vi "BMark_Create Tree.vi"(7 "Bookmarks":T2[](array[typedef]), 8 "Error In":errorcluster, 10 "Bookmarks Grouping":T1, 11 "Bookmarks View In":refnum<vi>) -> (0 "Error Out":errorcluster, 3 "Bookmarks View Out":refnum<vi>)   [LabVIEW 2018, in "Bookmark Manager.lvlib"]
uses:
  Bookmark Manager.lvlib
  Controls/BMark_Bookmark Data.ctl
  Controls/BMark_VI_Identifier.ctl
  <vilib>/addons/analyzer/_analyzerctrls.llb/VIAnCtl Analysis App Info.ctl
  Controls/Bookmarks Groups.ctl
  Toolkit/Typedefs/Bookmark Tags.ctl
  Toolkit/Toolkit.lvlib
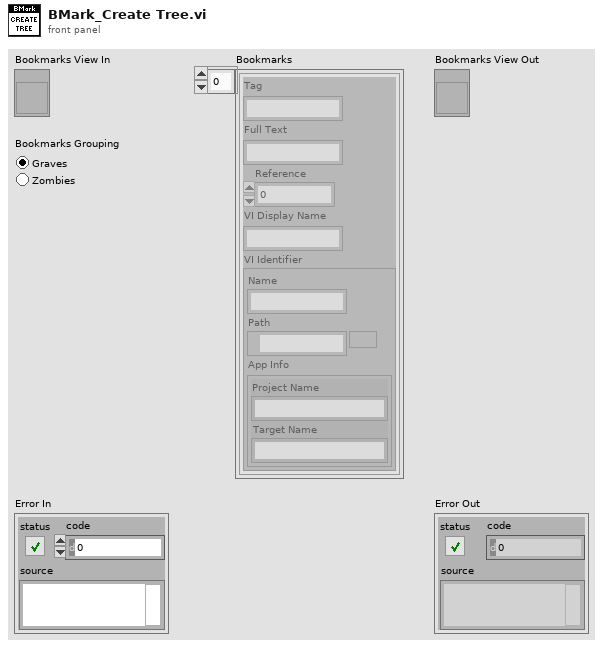
[diagram p1: front panel]
types:
  T1 = typedef "Bookmark Manager.lvlib/Bookmarks Groups.ctl" = enum32{"Graves", "Zombies"}
  T2 = typedef "Bookmark Manager.lvlib/BMark_Bookmark Data.ctl" = cluster{"Tag":string, "Full Text":string, "Reference":i32, "VI Display Name":string, "VI Identifier":T3}
  T3 = typedef "Bookmark Manager.lvlib/BMark_VI_Identifier.ctl" = cluster{"Name":string, "Path":path, "App Info":T4}
  T4 = typedef "VIAnCtl Analysis App Info.ctl" = cluster{"Project Name":string, "Target Name":string}
  T5 = enum8{"Enabled", "Disabled", "Disabled and Grayed Out"}
  T6 = typedef "Toolkit.lvlib/Bookmark Tags.ctl" = enum16{"RIP", "Zombie"}
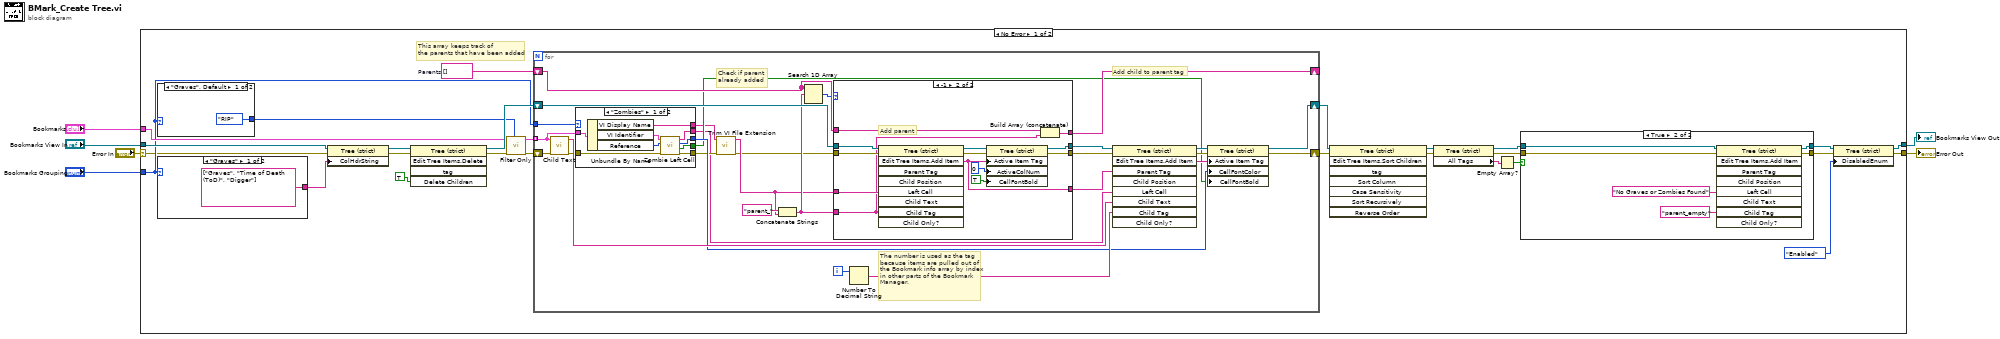
[diagram p0: block diagram]
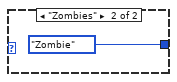
[diagram p2: hidden frame]
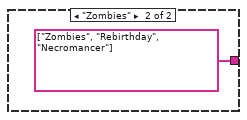
[diagram p3: hidden frame]
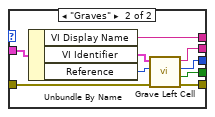
[diagram p4: hidden frame]
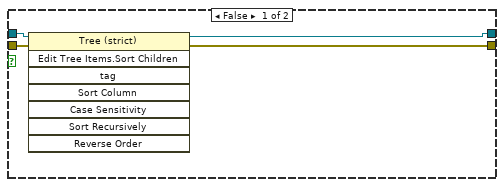
[diagram p6: hidden frame]
diagram:
  n1 = case shown="No Error" "Error In" {
    selector: "Error In" -> [w7 w112]
    tunnel: "Bookmarks View In" -> [w27 w111]
    tunnel: [w17 w112] -> w5
    tunnel: [w15 w111] -> w4
    tunnel: "Bookmarks" -> [w13 _]
    tunnel: "Bookmarks Grouping" -> [w8 _]
    frame No Error {
      w31 = string[] []  # Parents
      # "This array keeps track of \nthe parents that have been added"
      n2 = case shown="\"Graves\", Default" w8 {
        tunnel: [Bookmark_Tags."RIP" ("Bookmark") Bookmark_Tags."Zombie" ("Bookmark")] -> w12
        frame "Graves", Default {
        }
        frame "Zombies" {
        }
      }
      n3 = case shown="\"Graves\"" w8 {
        tunnel: [string[] ["Graves", "Time of Death (ToD)", "Digger"] string[] ["Zombies", "Rebirthday", "Necromancer"]] -> w14
        frame "Graves" {
        }
        frame "Zombies" {
        }
      }
      n4 = property class="Tree (strict)"(reference=w27, error in=w7, "ColHdrString"=w14) -> (reference out=w25:refnum<vi>, error out=w26:errorcluster)
      n5 = invoke class="Tree (strict)" method="Edit Tree Items.Delete"(reference=w25, error in=w26, "Delete Children"=TRUE ("Delete Children?")) -> (reference out=w32:refnum<vi>, error out=w11:errorcluster)  [unwired: 2 in, 3 out]
      n6 = call "Filter Only.vi"("Bookmark"=w12, "Error In"=w11, "All Bookmarks"=w13) -> ("Error Out"=w10:errorcluster, "Filtered Bookmarks"=w9:T2[])  [unwired: 7 in]
      n7 = for {
        tunnel: w9 -> [w52] mode=indexing
        shift-right: [w64] -> _
        shift-left: w31 -> [w65]
        shift-right: [w48] -> w30
        shift-left: w32 -> [w63]
        tunnel: w8 -> [w56]
        shift-right: [w46] -> w16
        shift-left: w10 -> [w51]
        i -> [w54]
        # "The number is used as the tag because items are pulled out of the Bookmark info array by index in other parts of the Bookmark Manager."
        # "Check if parent\nalready added"
        # "Add child to parent tag"
        n8 = call "Child Text.vi"("Error In"=w51, "Bookmark"=w52) -> ("Error Out"=w49:errorcluster, "Child Text"=w50:string[])  [unwired: 8 in]
        n9 = case shown="\"Zombies\"" w56 {
          tunnel: w52 -> [w74 w81]
          tunnel: [w73 w83] -> w39
          tunnel: [w68 w75] -> w38
          tunnel: w49 -> [w72 w82]
          tunnel: [w69 w78] -> w41
          tunnel: [w67 w76] -> w44
          tunnel: [w66 w77] -> w43
          frame "Zombies" {
            n10 = Unbundle By Name(w74) -> ("VI Display Name"=w73:string, "VI Identifier"=w71:T3, "Reference"=w70:i32)
            n11 = call "Zombie Left Cell.vi"("Error In"=w72, "Bookmark ID"=w70, "VI Identifier"=w71) -> ("Error Out"=w69:errorcluster, "Bold?"=w66:bool, "Color"=w67:u32, "Text"=w68:string)  [unwired: 5 in]
          }
          frame "Graves" {
            n12 = Unbundle By Name(w81) -> ("VI Display Name"=w83:string, "VI Identifier"=w80:T3, "Reference"=w79:i32)
            n13 = call "Grave Left Cell.vi"("Error In"=w82, "Bookmark ID"=w79, "VI Identifier"=w80) -> ("Error Out"=w78:errorcluster, "Bold?"=w77:bool, "Color"=w76:u32, "Text"=w75:string)  [unwired: 5 in]
          }
        }
        n14 = call "Trim VI File Extension.vi"("Error In"=w41, "VI File Name"=w39) -> ("Error Out"=w40:errorcluster, "VI Name"=w42:string)  [unwired: 8 in]
        n15 = Concatenate Strings("parent_", w42) -> (w58:string)
        n16 = Search 1D Array(1D array=w65, element=w58) -> (index of element=w55:i32)  [unwired: 1 in]
        n17 = case shown="-1" w55 {
          tunnel: w65 -> [w87 w100]
          tunnel: w58 -> [w84 w93]
          tunnel: [w87 w99] -> w64
          tunnel: w40 -> [w85 w97]
          tunnel: [w85 w90] -> w57
          tunnel: w63 -> [w86 w98]
          tunnel: [w86 w89] -> w62
          tunnel: [w84 w88] -> w61
          tunnel: w42 -> [_ w96]
          frame Default {
            # "Tag previously added"
          }
          frame -1 {
            # "Add parent"
            n18 = invoke class="Tree (strict)" method="Edit Tree Items.Add Item"(reference=w98, error in=w97, "Left Cell"=w96, "Child Tag"=w93) -> (reference out=w95:refnum<vi>, error out=w94:errorcluster, "Edit Tree Items:Add Item"=w88:string)  [unwired: 5 in, 6 out]
            n19 = property class="Tree (strict)"(reference=w95, error in=w94, "Active Item Tag"=w88, "ActiveColNum"=0 ("Active Cell:Active Column Number"), "CellFontBold"=TRUE ("Active Cell:Cell Font:Bold")) -> (reference out=w89:refnum<vi>, error out=w90:errorcluster)
            n20 = Build Array (concatenate)(w100, w93) -> (w99:string[])
          }
        }
        n21 = Number To Decimal String(number=w54) -> (decimal integer string=w53:string)  [unwired: 1 in]
        n22 = invoke class="Tree (strict)" method="Edit Tree Items.Add Item"(reference=w62, error in=w57, "Parent Tag"=w61, "Left Cell"=w38, "Child Text"=w50, "Child Tag"=w53) -> (reference out=w59:refnum<vi>, error out=w47:errorcluster, "Edit Tree Items:Add Item"=w45:string)  [unwired: 3 in, 6 out]
        n23 = property class="Tree (strict)"(reference=w59, error in=w47, "Active Item Tag"=w45, "CellFontColor"=w44, "CellFontBold"=w43) -> (reference out=w48:refnum<vi>, error out=w46:errorcluster)
      }
      n24 = invoke class="Tree (strict)" method="Edit Tree Items.Sort Children"(reference=w30, error in=w16) -> (reference out=w24:refnum<vi>, error out=w23:errorcluster)  [unwired: 6 in, 6 out]
      n25 = property class="Tree (strict)"(reference=w24, error in=w23) -> (reference out=w29:refnum<vi>, error out=w28:errorcluster, "All Tags"=w22:string[])
      n26 = Empty Array?(array=w22) -> (empty?=w21:bool)
      n27 = case shown="True" w21 {
        tunnel: w29 -> [w104 w110]
        tunnel: w28 -> [w103 w109]
        tunnel: [w102 w108] -> w19
        tunnel: [w101 w106] -> w20
        frame False {
          n28 = invoke class="Tree (strict)" method="Edit Tree Items.Sort Children"(reference=w104, error in=w103) -> (reference out=w101:refnum<vi>, error out=w102:errorcluster)  [unwired: 6 in, 6 out]
        }
        frame True {
          n29 = invoke class="Tree (strict)" method="Edit Tree Items.Add Item"(reference=w110, error in=w109, "Left Cell"="No Graves or Zombies Found", "Child Tag"="parent_empty") -> (reference out=w106:refnum<vi>, error out=w108:errorcluster)  [unwired: 5 in, 7 out]
        }
      }
      n30 = property class="Tree (strict)"(reference=w20, error in=w19, "DisabledEnum"=T5."Enabled" ("Disabled")) -> (reference out=w15:refnum<vi>, error out=w17:errorcluster)
    }
    frame Error {
    }
  }
  "Error Out" <- w5
  "Bookmarks View Out" <- w4
